vi "Get DB Record.vi"(8 "error in (no error)":errorcluster, 10 "Record":T1 {"Balance" format="%_4p"}, 11 "ATM Controller in":refnum<class "ATM Controller.lvclass">) -> (0 "error out":errorcluster, 3 "ATM Controller out":refnum<class "ATM Controller.lvclass">)   [LabVIEW 2019, in "ATM Controller.lvlib" / "ATM Controller.lvclass"]
uses:
  ATM Controller.lvclass
  Simulated Configuration Database Actor/Simulated Configuration Database Actor/Records -cluster.ctl
  ATM Controller.lvclass/ATM Controller.ctl
  Simulated Configuration Database Actor/Simulated Configuration Database Actor/Configuration Database Actor.lvclass
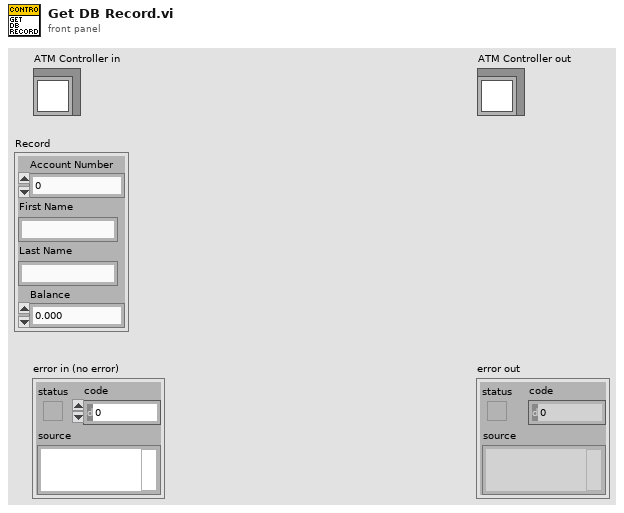
[diagram p1: front panel]
types:
  T1 = typedef "Configuration Database Actor.lvlib/Configuration Database Actor.lvclass/Records -cluster.ctl" = cluster{"Account Number":i32, "First Name":string, "Last Name":string, "Balance":i32}
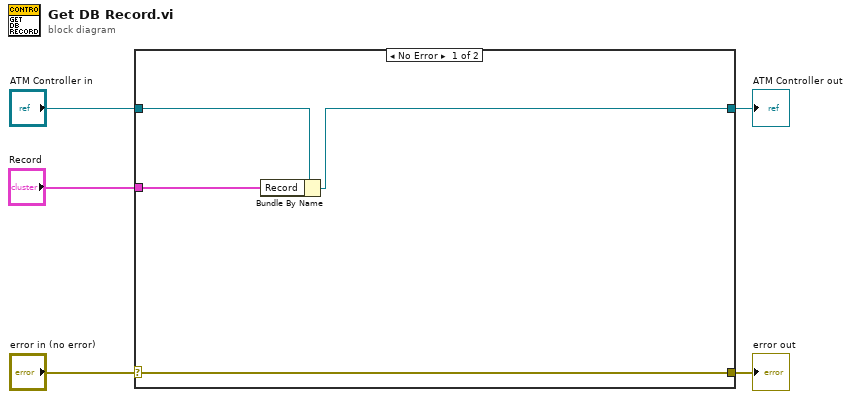
[diagram p0: block diagram]
diagram:
  n1 = case shown="No Error" "error in (no error)" {
    selector: "error in (no error)" -> [w9 w11]
    tunnel: [w9 w11] -> w4
    tunnel: [w7 w10] -> w2
    tunnel: "ATM Controller in" -> [w8 w10]
    tunnel: "Record" -> [w6 _]
    frame No Error {
      n2 = Bundle By Name(cluster=w8, "Record"=w6) -> (w7:refnum<class "ATM Controller.lvclass">)
    }
    frame Error {
    }
  }
  "error out" <- w4
  "ATM Controller out" <- w2
